vi "myRIO_BRig_RT_dataExp_TPB_min__R.vi"() -> (2 "output_TPB_min__R":i32)   [LabVIEW 2014]
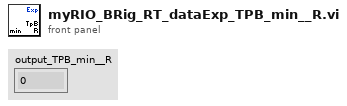
[diagram p1: front panel]
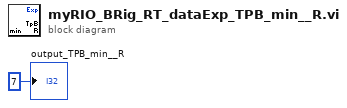
[diagram p0: block diagram]
diagram:
  "output_TPB_min__R" <- 7 ("output_iBlock")
